vi "From BananaLeaf.TestSuite.vi"(11 "Leaf.Properties.TestSuite":refnum<class "Leaf.Properties.Suite.lvclass">) -> (2 "Properties.Suite":refnum<class "Properties.Suite.lvclass">)   [LabVIEW 2021, in "Banana.Caraya.lvlib" / "Leaf.Properties.Suite.lvclass"]
uses:
  Leaf.Properties.Suite.lvclass
  C:/Repositories/LVOS/Bananas/lv-src/Banana.Caraya/Leaf.Properties/Leaf.Properties.lvclass
  <vilib>/addons/_JKI Toolkits/Caraya/classes/Properties.Suite/Properties.Suite.lvclass
  Leaf.Properties/Leaf.Properties.lvclass/Leaf.Properties.ctl
  Leaf.Properties.Suite.lvclass/Leaf.Properties.Suite.ctl
  Leaf.Properties/Leaf.Properties.lvclass
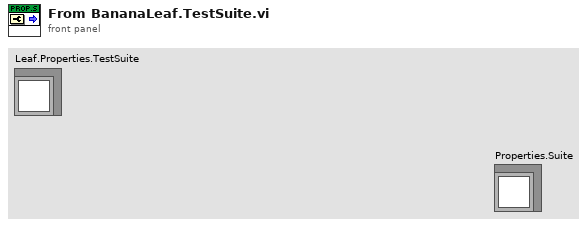
[diagram p1: front panel]
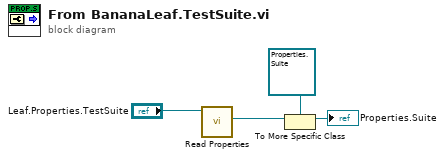
[diagram p0: block diagram]
diagram:
  n1 = call "Read Properties.vi"("Leaf.Properties in"="Leaf.Properties.TestSuite") -> ("Properties"=w3:refnum<class "Properties.lvclass">)  [unwired: 9 in, 1 out]
  n2 = To More Specific Class(target class=refnum<class "Properties.Suite.lvclass"> refnum ("Properties.Suite"), reference=w3) -> (specific class reference=→"Properties.Suite":refnum<class "Properties.Suite.lvclass">)  [unwired: 1 in, 1 out]
